vi "Simple Test.vi"() -> ()   [LabVIEW 2016]
uses:
  src/Typedefs/Interpolation Configuration--cluster.ctl
  src/subVIs/Get X and Y (single).vi
  <vilib>/Analysis/baseanly.llb/Mean.vi
  <vilib>/Analysis/baseanly.llb/Mean (DBL).vi
  src/XY to 2D.vi
  <userlib>/LevyLab/Control VI/Other/Ramp_SubVI.vi
  src/xy_utilities.lvlib
panel:
  out "size(s) 2":i32
  out "size(s)":i32
  out "execution time (s)":dbl
  out "XY Data 2":cluster{"X-array":dbl[], "Y-array":dbl[]}(graph)
  out "XY Data":cluster{"X-array":dbl[], "Y-array":dbl[]}[](graph)
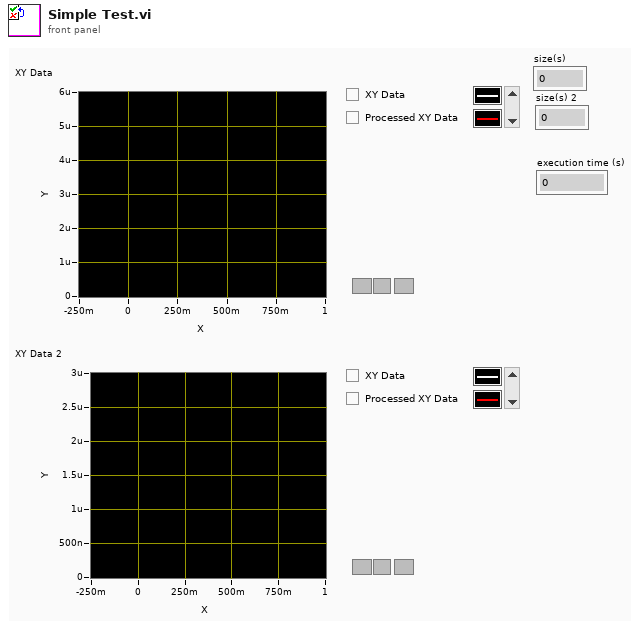
[diagram p1: front panel]
types:
  T1 = typedef "xy_utilities.lvlib/Interpolation Configuration--cluster.ctl" = cluster{"X Low":dbl, "X High":dbl, "X Step":dbl, "Fake Point":dbl}
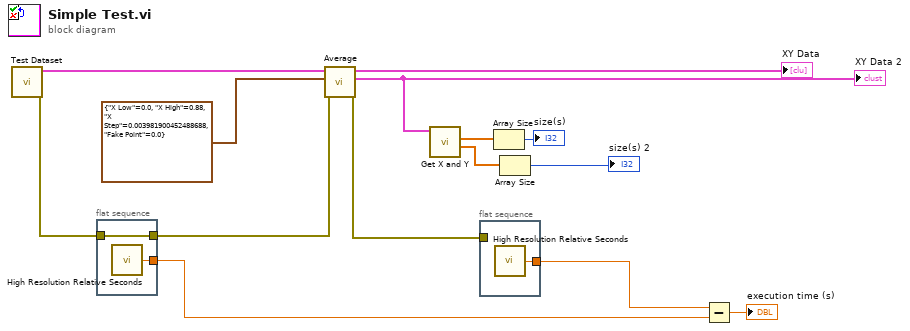
[diagram p0: block diagram]
diagram:
  n1 = call "Test Dataset.vi"() -> ("error out"=w11:errorcluster, "XY-data out"=w14:cluster{"X-array":dbl[], "Y-array":dbl[]}[])  [unwired: 9 in, 1 out]
  n2 = flat-sequence {
    tunnel: [w16] -> w12
    tunnel: w11 -> [w16]
    tunnel: [w15] -> w8
    frame #0 {
      n3 = call <vilib>:"High Resolution Relative Seconds.vi"() -> ("relative seconds"=w15:dbl)
    }
  }
  n4 = call "Average.vi"("error in (no error)"=w12, "Configure"=T1 {"X Low"=0.0, "X High"=0.88, "X Step"=0.003981900452488688, "Fake Point"=0.0}, "XY-data"=w14) -> ("error out"=w10:errorcluster, "Averaged XY-data out"=w6:cluster{"X-array":dbl[], "Y-array":dbl[]}, "XY-data out"=→"XY Data":cluster{"X-array":dbl[], "Y-array":dbl[]}[])  [unwired: 6 in]
  "XY Data 2" <- w6
  n5 = call-poly "Get X and Y.vi"("XY-data"=w6) -> ("Y-array"=w4:dbl[], "X-array"=w5:dbl[])  [unwired: 7 in, 2 out]
  n6 = flat-sequence {
    tunnel: w10 -> [_]
    tunnel: [w17] -> w9
    frame #0 {
      n7 = call <vilib>:"High Resolution Relative Seconds.vi"() -> ("relative seconds"=w17:dbl)
    }
  }
  n8 = Array Size(array=w5) -> (size(s)=→"size(s)":i32)
  n9 = Array Size(array=w4) -> (size(s)=→"size(s) 2":i32)
  n10 = Subtract(x=w9, y=w8) -> (x-y=→"execution time (s)":dbl)
